vi "1 colum data.vi"(9 "column":string, 10 "table":string, 11 "Refnum in":T1) -> (1 "data":string[](array[string]), 2 "table":string, 3 "Refnum out":T1)   [LabVIEW 2017]
uses:
  <vilib>/addons/database/Connection.llb/Conn ObjectReference.ctl
  <vilib>/addons/database/Connection.llb/Conn Execute.vi
  <vilib>/addons/database/Recordset.llb/Rec Fetch Recordset Data (R).vi
  <vilib>/addons/database/Recordset.llb/Rec Destroy - Connection.vi
  <vilib>/addons/database/_DB Variant To Data/Database Variant To Data.xnode
  <vilib>/addons/database/NI_Database_API.lvlib
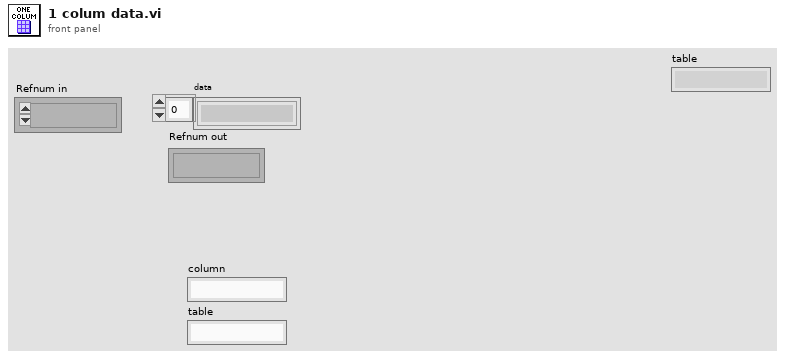
[diagram p1: front panel]
types:
  T1 = typedef "NI_Database_API.lvlib/Conn ObjectReference.ctl" = refnum<k1>
  T2 = typedef "NI_Database_API.lvlib/Rec ObjectReference.ctl" = refnum<k1>
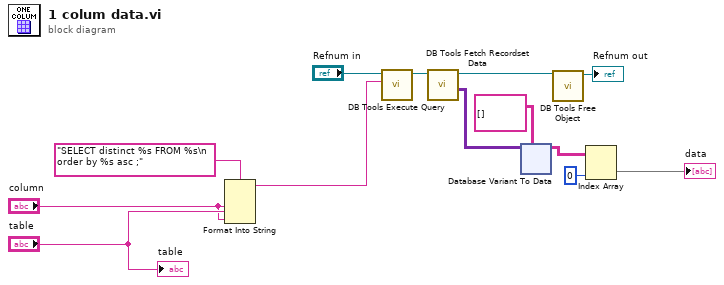
[diagram p0: block diagram]
diagram:
  n1 = Format Into String(format string="SELECT distinct %s FROM %s\n order by %s asc ;" ("SQL query"), "column", "table", "column") -> (resulting string=w3:string)  [unwired: 2 in, 1 out]
  n2 = call-poly <vilib>:"DB Tools Execute Query.vi"("SQL query"=w3, "connection reference"="Refnum in") -> ("recordset reference"=w6:T2)  [unwired: 6 in, 1 out]
  n3 = call-poly <vilib>:"DB Tools Fetch Recordset Data.vi"("recordset reference"=w6) -> ("recordset data"=w9:variant[][], "recordset reference out"=w8:T2)  [unwired: 4 in, 1 out]
  n4 = xnode "Database Variant To Data"("database variant"=w9, "type"=string[][] []) -> ("data"=w11:string[][])  [unwired: 1 in, 1 out]
  n5 = call-poly <vilib>:"DB Tools Free Object.vi"("recordset reference"=w8) -> ("connection reference"=→"Refnum out":T1)  [unwired: 9 in, 1 out]
  n6 = Index Array(array=w11, index (col)=0 ("disabled index (col)")) -> (element=→"data":string[])  [unwired: 1 in]
  "table" <- "table"
